vi "rt_cdmockup_StateMachine.vi"() -> ()   [LabVIEW 2020]
uses:
  <vilib>/NI VeriStand/Custom Device API/Hardware Interface Driver VI Operation.ctl
  <vilib>/NI VeriStand/Custom Device API/Custom Device Item Ref.ctl
  <vilib>/Platform/TimedLoop/XDataNode/timing_clust.ctl
  <vilib>/Platform/TimedLoop/XDataNode/nitl_modes.ctl
  <vilib>/Platform/TimedLoop/XDataNode/wakeup.ctl
  Source/RT Driver/RT Driver VI.vi
  <vilib>/platform/TimedLoop/XDataNode/XDataNode.xnode
  <vilib>/Platform/TimedLoop/XDataNode/XDNodeRunTimeDep.lvlib
  Source/RT Driver/Ballard MIL-1553 Engine.lvlib
  <vilib>/NI VeriStand/Custom Device API/Custom Device API.lvlib
panel:
  in  "Loop rate uS":i64=10000
  out "action count":i32
  out "Error Code":i32
  in  "Device Reference in":T1=18446744073709551615 format="%.0x"
  in  "Operation":T2
  out "error out":errorcluster
  in  "stop":bool
  in  "Run Action":bool
  # "!!!IMPORTANT: set RtDriverMockupMode and debug conditional disable\nsymbols to True to run it effectively!! Then read contents of the errlog.txt file to see print debugs\n\n clear && tail -f /var/local/natinst/log/errlog.txt"
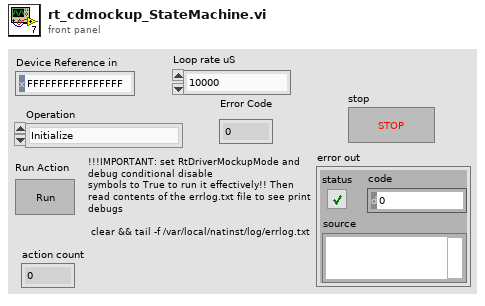
[diagram p1: front panel]
types:
  T1 = typedef "Custom Device API.lvlib/Custom Device Item Ref.ctl" = u64
  T2 = typedef "Custom Device API.lvlib/Hardware Interface Driver VI Operation.ctl" = enum16{"Initialize", "Start", "Read Data from HW", "Write Data to HW", "Close"}
  T3 = typedef "XDNodeRunTimeDep.lvlib/timing_clust.ctl" = cluster{"Expected End [f-1]":u64, "Actual End [f-1]":u64, "Finished Late? [f-1]":bool, "Expected End [i-1]":u64, "Actual End [i-1]":u64, "Finished Late? [i-1]":bool, "Expected Start [i]":u64, "Actual Start [i]":u64, "Expected Start [f]":u64, "Actual Start [f]":u64, "Source Name":string, "Structure Name":string, "Period":i64, "Deadline":i64, "Offset":i64, "Start":i64, "Priority":i32, "Timeout":i32, "Mode":T4, "Wakeup Reason":T5, "Error":errorcluster, "Source Type":string, "Secondary Source Type":string, "Global End Time":u64, "Global Start Time":u64, "Frame Duration":u64, "Iteration Duration":u64, "Assigned CPU":i32, "I/O Scan Engine Mode":u32}
  T4 = typedef "XDNodeRunTimeDep.lvlib/nitl_modes.ctl" = enum32{"No Change", "Process missed periods, maintain original phase", "Discard missed periods, maintain original phase", "Process missed periods, ignore original phase", "Discard missed periods, ignore original phase"}
  T5 = typedef "XDNodeRunTimeDep.lvlib/wakeup.ctl" = enum32{"Normal", "Aborted", "Asynchronous wakeup", "Timing source error", "Timed loop error", "Timeout"}
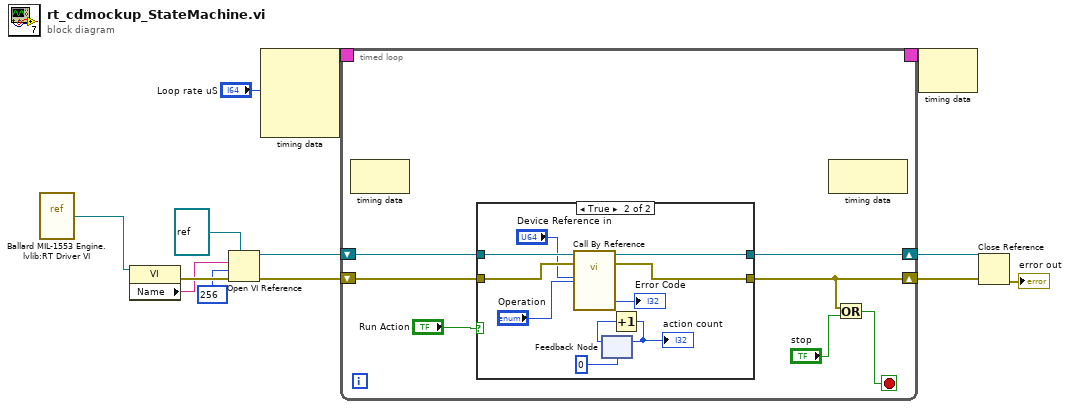
[diagram p0: block diagram]
diagram:
  n1 = vi-ref "Ballard MIL-1553 Engine.lvlib:RT Driver VI.vi"() -> (w9:refnum<vi>)
  n2 = property class="VI"(reference=w9) -> (error out=w12:errorcluster, "Name"=w11:string)  [unwired: 1 in, 1 out]
  n3 = Open VI Reference(type specifier VI Refnum (for type only)=refnum<vi> refnum, vi path=w11, options=256, error in (no error)=w12) -> (vi reference=w8:refnum<vi>, error out=w7:errorcluster)  [unwired: 2 out]
  n4 = node-c288("Loop rate uS") -> (w3:T3)  [unwired: 3 in]
  n5 = timed-loop {
    shift-right: [w18] -> w5
    shift-left: w8 -> [w19]
    shift-right: [w14] -> w6
    shift-left: w7 -> [w17]
    timing: w3 -> [_]
    timing-out: [_] -> w2
    stop <- w15 stop-if-true
    n6 = node-c288() -> ()  [unwired: 1 in, 1 out]
    n7 = case shown="True" "Run Action" {
      tunnel: w19 -> [w24 w34]
      tunnel: [w24 w32] -> w18
      tunnel: w17 -> [w23 w33]
      tunnel: [w23 w31] -> w14
      frame False {
      }
      frame True {
        n8 = call-by-ref "?"(reference=w34, error in=w33, "Operation"="Operation", "Device Reference in"="Device Reference in") -> (reference out=w32:refnum<vi>, error out=w31:errorcluster, "Error Code"=→"Error Code":i32)  [unwired: 9 in]
        n9 = feedback #1(0) -> (w27:i32)
        n10 = Increment(x=w27) -> (x+1=w26:i32)
        "action count" <- w26
        n11 = feedback-in #1(w26) -> ()
      }
    }
    n12 = node-c288() -> ()  [unwired: 1 in, 1 out]
    n13 = Or(x=w14, y="stop") -> (x .or. y?=w15:bool)
  }
  n14 = node-c288(w2) -> ()  [unwired: 1 out]
  n15 = Close Reference(reference=w5, error in (no error)=w6) -> (error out=→"error out":errorcluster)
